vi "Symphony Acquire Spectrum Clean.vi"(5 "Acquire":refnum<vi>, 7 "Running":refnum<vi>, 8 "error in":errorcluster caption="Error In", 10 "ShutterOpen":bool, 11 "JYCCDLib.IJYCCDReqd":refnum<k7>) -> (0 "Acq Time(ms)":u32, 3 "Raw Data":i32[][](array[numeric]))   [LabVIEW 2010]
panel:
  out "ReadyForAcquisition":bool
  out "Data":i32[][](graph)
  out "AcquisitionBusy":bool
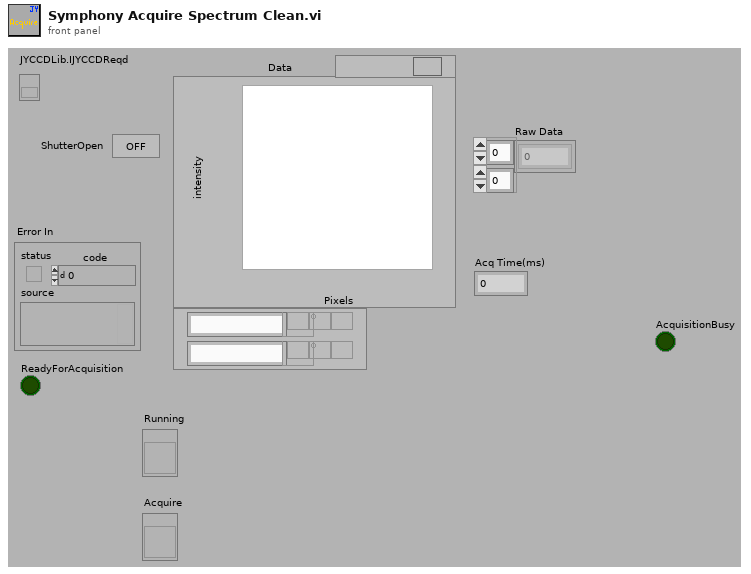
[diagram p1: front panel]
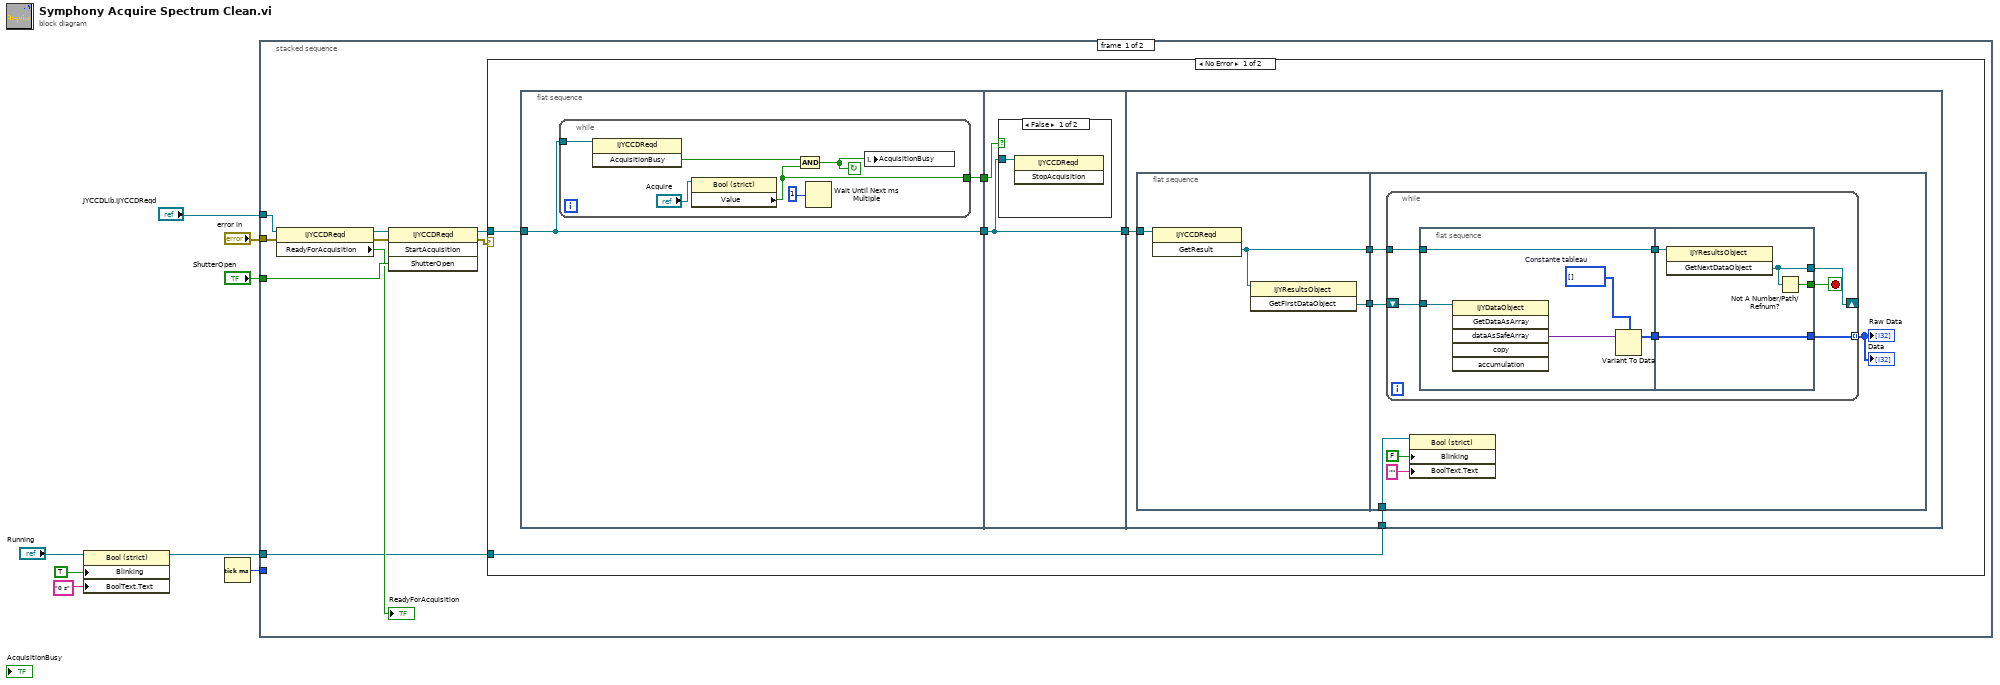
[diagram p0: block diagram]
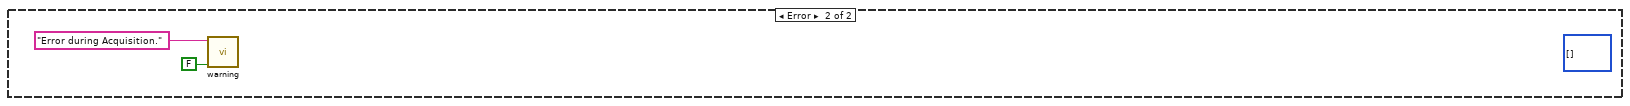
[diagram p3: hidden frame]
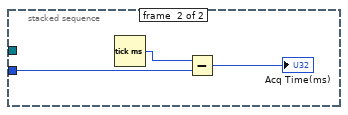
[diagram p4: hidden frame]
diagram:
  n1 = property class="Bool (strict)"(reference="Running", "Blinking"=TRUE ("Blinkend"), "BoolText.Text"="0 s" ("Boolean Text.Text")) -> (reference out=w1:refnum<vi>)  [unwired: 1 in, 1 out]
  n2 = Tick Count (ms)() -> (millisecond timer value=w5:u32)
  n3 = stacked-sequence {
    tunnel: "JYCCDLib.IJYCCDReqd" -> [w16 _]
    tunnel: "error in" -> [w15 _]
    tunnel: "ShutterOpen" -> [w17 _]
    tunnel: w5 -> [_ w65]
    tunnel: w1 -> [w9 _]
    frame #0 {
      n4 = property class="IJYCCDReqd"(reference=w16, error in=w15) -> (reference out=w14:refnum<k7>, error out=w13:errorcluster, "ReadyForAcquisition"=→"ReadyForAcquisition":bool)
      n5 = invoke class="IJYCCDReqd" method="StartAcquisition"(reference=w14, error in=w13, "ShutterOpen"=w17) -> (reference out=w10:refnum<k7>, error out=w11:errorcluster)  [unwired: 1 in, 2 out]
      n6 = case shown="No Error" w11 {
        tunnel: w10 -> [w22 _]
        tunnel: w9 -> [w18 _]
        frame No Error {
          n7 = flat-sequence {
            tunnel: w22 -> [w24]
            tunnel: [w24] -> w21
            tunnel: [w23] -> w19
            tunnel: w21 -> [w32]
            tunnel: [w32] -> w20
            tunnel: w19 -> [w31]
            tunnel: w20 -> [w37]
            tunnel: w18 -> [w34]
            frame #0 {
              n8 = while {
                tunnel: w24 -> [w30]
                tunnel: [w25] -> w23
                stop <- w27 continue-if-true
                n9 = invoke class="IJYCCDReqd" method="AcquisitionBusy"(reference=w30) -> ("AcquisitionBusy"=w28:bool)  [unwired: 2 in, 2 out]
                n10 = property class="Bool (strict)"(reference="Acquire") -> ("Value"=w25:bool)  [unwired: 1 in, 2 out]
                n11 = And(x=w28, y=w25) -> (x .and. y?=w27:bool)
                n12 = Wait Until Next ms Multiple(millisecond multiple=u32 1 ("n millisecondes")) -> ()  [unwired: 1 out]
                n13 = local write "AcquisitionBusy"(w27) -> ()
              }
            }
            frame #1 {
              n14 = case shown="False" w31 {
                tunnel: w32 -> [w33 _]
                frame False {
                  n15 = invoke class="IJYCCDReqd" method="StopAcquisition"(reference=w33) -> ()  [unwired: 2 in, 3 out]
                }
                frame True {
                }
              }
            }
            frame #2 {
              n16 = flat-sequence {
                tunnel: w37 -> [w40]
                tunnel: [w39] -> w36
                tunnel: [w38] -> w35
                tunnel: w36 -> [w46]
                tunnel: w35 -> [w45]
                tunnel: w34 -> [w41]
                frame #0 {
                  n17 = invoke class="IJYCCDReqd" method="GetResult"(reference=w40) -> ("GetResult"=w39:refnum<k7>)  [unwired: 2 in, 2 out]
                  n18 = invoke class="IJYResultsObject" method="GetFirstDataObject"(reference=w39) -> ("GetFirstDataObject"=w38:refnum<k7>)  [unwired: 2 in, 2 out]
                }
                frame #1 {
                  n19 = while {
                    tunnel: [w50] -> w44 mode=indexing
                    tunnel: w46 -> [w52]
                    shift-left: w45 -> [w53]
                    shift-right: [w51] -> _
                    stop <- w49 stop-if-true
                    n20 = flat-sequence {
                      tunnel: w53 -> [w57]
                      tunnel: w52 -> [w54]
                      tunnel: [w54] -> w48
                      tunnel: [w56] -> w47
                      tunnel: w48 -> [w62]
                      tunnel: [w61] -> w51
                      tunnel: [w59] -> w50
                      tunnel: w47 -> [w59]
                      tunnel: [w60] -> w49
                      frame #0 {
                        w55 = i32[] []  # Constante tableau
                        n21 = invoke class="IJYDataObject" method="GetDataAsArray"(reference=w57) -> ("dataAsSafeArray"=w58:variant)  [unwired: 5 in, 5 out]
                        n22 = Variant To Data(Variant=w58, type=w55) -> (data=w56:i32[])  [unwired: 1 in, 1 out]
                      }
                      frame #1 {
                        n23 = invoke class="IJYResultsObject" method="GetNextDataObject"(reference=w62) -> ("GetNextDataObject"=w61:refnum<k7>)  [unwired: 2 in, 2 out]
                        n24 = Not A Number/Path/Refnum?(number/path/refnum=w61) -> (NaN/Path/Refnum?=w60:bool)
                      }
                    }
                  }
                  "Data" <- w44
                  "Raw Data" <- w44
                  n25 = property class="Bool (strict)"(reference=w41, "Blinking"=FALSE ("Blinkend"), "BoolText.Text"="" ("Boolean Text.Text")) -> ()  [unwired: 1 in, 2 out]
                }
              }
            }
          }
        }
        frame Error {
          (unwired) i32[][] [] ("type")
          n26 = call "warning.vi"("with cancel ?"=FALSE, "Text"="Error during Acquisition.") -> ()  [unwired: 2 in, 1 out]
        }
      }
    }
    frame #1 {
      n27 = Tick Count (ms)() -> (millisecond timer value=w66:u32)
      n28 = Subtract(x=w66, y=w65) -> (x-y=→"Acq Time(ms)":u32)
    }
  }
